vi "Set LV Color.vi"(8 "error in (no error)":errorcluster, 10 "Color (black)":u32(colorbox), 11 "Color in":refnum<class "Color.lvclass">) -> (0 "error out":errorcluster, 3 "Color out":refnum<class "Color.lvclass">)   [LabVIEW 2018, in "Color.lvclass"]
doc: "A method to set the color from a LabVIEW color value. If the same color cannot be shown in the color model, the closest color will be selected."
uses:
  Color.lvclass
panel:
  # "expressionflow.com"
  # "Copyright (c) 2008 Tomi Maila. All rights reserved."
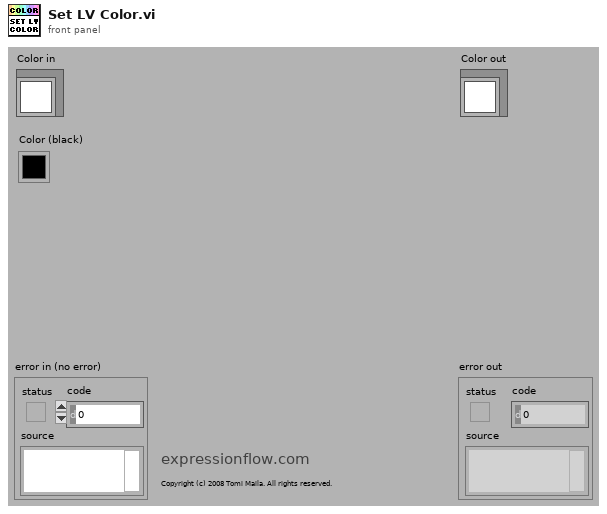
[diagram p1: front panel]
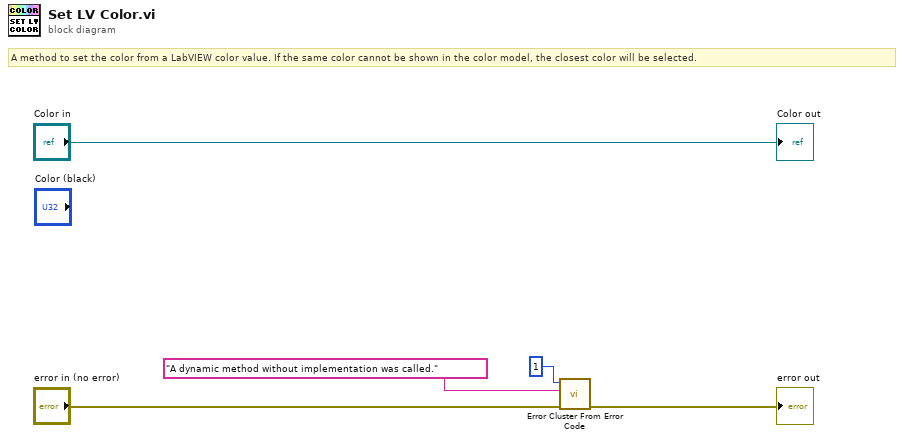
[diagram p0: block diagram]
diagram:
  # "A method to set the color from a LabVIEW color value. If the same color cannot be shown in the color model, the closest color will be selected."
  n1 = call <vilib>:"Error Cluster From Error Code.vi"("error in (no error)"="error in (no error)", "error message (\"\")"="A dynamic method without implementation was called." ("error message (\"\")"), "error code (0)"=1) -> ("error out"=→"error out":errorcluster)  [unwired: 6 in]
  "Color out" <- "Color in"
